vi "APS home move.vi"(8 "error in (no error)":errorcluster caption="错误输入（无错误）", 11 "Axis_ID":i32) -> (0 "error out":errorcluster caption="错误输出", 3 "function return":i32)   [LabVIEW 2012, in "APS168.lvlib"]
doc: "I32 FNTYPE APS_home_move( I32 Axis_ID );"
uses:
  APS168.lvlib
  Global/global.vi
  APS168.dll
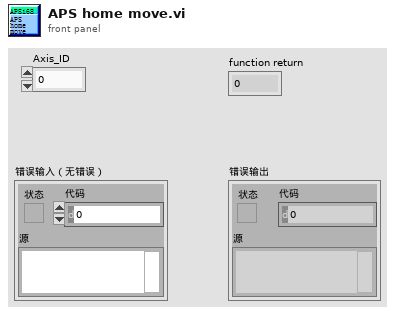
[diagram p1: front panel]
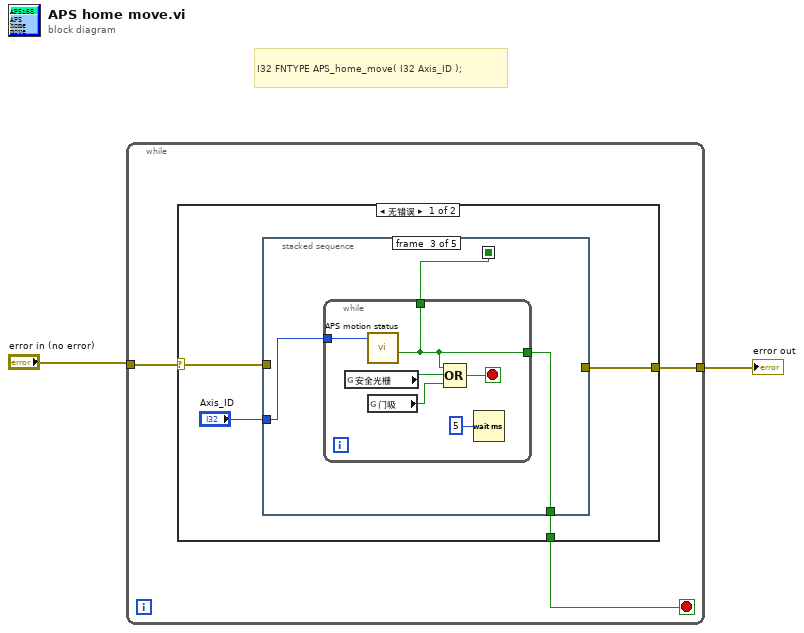
[diagram p0: block diagram]
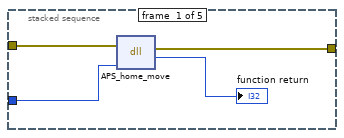
[diagram p2: hidden frame]
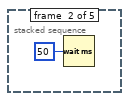
[diagram p3: hidden frame]
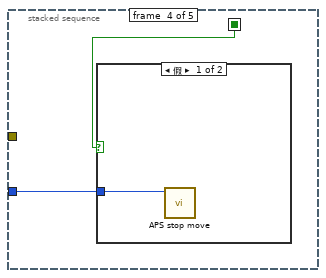
[diagram p4: hidden frame]
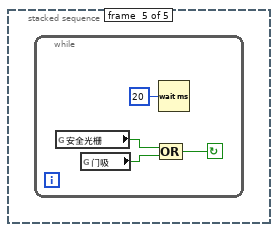
[diagram p6: hidden frame]
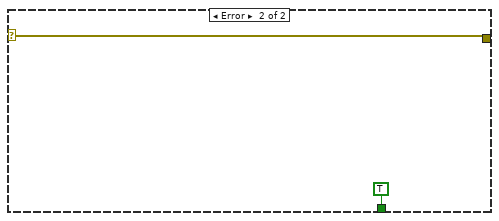
[diagram p7: hidden frame]
diagram:
  # "I32 FNTYPE APS_home_move( I32 Axis_ID );"
  n1 = while {
    tunnel: [w5] -> w2
    tunnel: "error in (no error)" -> [w4]
    stop <- w3 stop-if-true
    n2 = case shown="无错误" w4 {
      selector: w4 -> [w7 w32]
      tunnel: [w9 w32] -> w5
      tunnel: [w6 TRUE ("x与y?")] -> w3
      frame No Error {
        n3 = stacked-sequence {
          seq-local: [_ _ w15 _ _] -> [_ _ _ w25 _]
          tunnel: [w12 _ _ _ _] -> w9
          tunnel: "Axis_ID" -> [w11 _ w17 w24 _]
          tunnel: w7 -> [w10 _ _ _ _]
          tunnel: [_ _ w16 _ _] -> w6
          frame #0 {
            n4 = dll-call lib="PTH1/abs E\t冲压机LLB运动204cAPS168.*" fn="APS_home_move"(error in=w10, "Axis_ID"=w11) -> (error out=w12:errorcluster, "return type"=→"function return":i32)  [unwired: 3 in, 1 out]
          }
          frame #1 {
            n5 = Wait (ms)(milliseconds to wait=u32 50 ("等待时间（毫秒）")) -> ()  [unwired: 1 out]
          }
          frame #2 {
            n6 = while {
              tunnel: w17 -> [w22]
              tunnel: [w19] -> w16
              tunnel: [w19] -> w15
              stop <- w21 stop-if-true
              n7 = global read "global.vi" "安全光栅"() -> (w20:bool)
              n8 = call "APS motion status.vi"("Axis_ID"=w22) -> ("x与y?"=w19:bool)  [unwired: 9 in, 1 out]
              n9 = global read "global.vi" "门吸"() -> (w18:bool)
              n10 = Compound Arithmetic op=OR(w19, w20, w18) -> (w21:bool)
              n11 = Wait (ms)(milliseconds to wait=u32 5 ("等待时间（毫秒）")) -> ()  [unwired: 1 out]
            }
          }
          frame #3 {
            n12 = case shown="假" w25 {
              tunnel: w24 -> [w26 _]
              frame False {
                n13 = call "APS stop move.vi"("Axis_ID"=w26) -> ()  [unwired: 9 in, 2 out]
              }
              frame True {
              }
            }
          }
          frame #4 {
            n14 = while {
              stop <- w27 continue-if-true
              n15 = global read "global.vi" "安全光栅"() -> (w29:bool)
              n16 = global read "global.vi" "门吸"() -> (w28:bool)
              n17 = Wait (ms)(milliseconds to wait=u32 20 ("等待时间（毫秒）")) -> ()  [unwired: 1 out]
              n18 = Compound Arithmetic op=OR(w29, w28) -> (w27:bool)
            }
          }
        }
      }
      frame Error {
      }
    }
  }
  "error out" <- w2
